vi "Simple SysDef API_Poly.vi"   [LabVIEW 2019, in "Simple SysDef API.lvlib"]
uses:
  <userlib>/SimpleSysDef/Simple SysDef API.lvlib
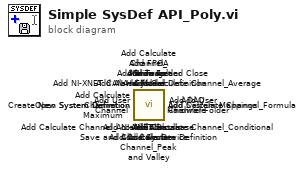
[diagram p0: block diagram]
diagram:
  n1 = call <userlib>:"Add NI-XNET Database.vi"() -> ()  [unwired: 9 in, 3 out]
  n2 = call <userlib>:"Save As and Close System Definition.vi"() -> ()  [unwired: 10 in, 2 out]
  n3 = call <userlib>:"Open System Definition.vi"() -> ()  [unwired: 9 in, 3 out]
  n4 = call <userlib>:"Add System Mappings.vi"() -> ()  [unwired: 10 in, 2 out]
  n5 = call <userlib>:"Add Custom Device.vi"() -> ()  [unwired: 9 in, 3 out]
  n6 = call <userlib>:"Add Model.vi"() -> ()  [unwired: 9 in, 3 out]
  n7 = call <userlib>:"Add Alias Folder.vi"() -> ()  [unwired: 9 in, 3 out]
  n8 = call <userlib>:"Add User Channel.vi"() -> ()  [unwired: 9 in, 3 out]
  n9 = call <userlib>:"Add User Channel Folder.vi"() -> ()  [unwired: 9 in, 3 out]
  n10 = call <userlib>:"Add Alias.vi"() -> ()  [unwired: 9 in, 3 out]
  n11 = call <userlib>:"Add Alarm.vi"() -> ()  [unwired: 9 in, 3 out]
  n12 = call <userlib>:"Add Alarm Folder.vi"() -> ()  [unwired: 9 in, 3 out]
  n13 = call <userlib>:"Add Calculate Channel_Conditional.vi"() -> ()  [unwired: 9 in, 3 out]
  n14 = call <userlib>:"Add Calculate Channel_Peak and Valley.vi"() -> ()  [unwired: 9 in, 3 out]
  n15 = call <userlib>:"Add Calculate Channel_Minimum.vi"() -> ()  [unwired: 9 in, 3 out]
  n16 = call <userlib>:"Add Calculate Channel_Maximum.vi"() -> ()  [unwired: 9 in, 3 out]
  n17 = call <userlib>:"Add Calculate Channel_Acceleration.vi"() -> ()  [unwired: 9 in, 3 out]
  n18 = call <userlib>:"Add Calculate Channel_Average.vi"() -> ()  [unwired: 9 in, 3 out]
  n19 = call <userlib>:"Add Calculate Channel_Formula.vi"() -> ()  [unwired: 9 in, 3 out]
  n20 = call <userlib>:"Add NI-XNET CAN Hardware.vi"() -> ()  [unwired: 9 in, 3 out]
  n21 = call <userlib>:"Add FPGA Hardware.vi"() -> ()  [unwired: 9 in, 3 out]
  n22 = call <userlib>:"Save and Close System Definition.vi"() -> ()  [unwired: 10 in, 2 out]
  n23 = call <userlib>:"Create New System Definition.vi"() -> ()  [unwired: 9 in, 3 out]
  n24 = call <userlib>:"Add DAQ Hardware.vi"() -> ()  [unwired: 9 in, 3 out]
  n25 = call <userlib>:"Add Chassis.vi"() -> ()  [unwired: 9 in, 3 out]
  n26 = call <userlib>:"Add Target.vi"() -> ()  [unwired: 9 in, 3 out]
